vi "gentec-M-Link.Set Anticipation.vi"(0 "VISA resource In":refnum<visa-resource-name>, 2 "Enable Anticipation":bool, 5 "error in (no error)":errorcluster) -> (11 "Data Read":string, 13 "Read Timeout":bool, 14 "VISA resource Out":refnum<visa-resource-name>, 16 "Success":bool, 19 "error out":errorcluster)   [LabVIEW 2014, in "gentec-M-Link - Driver.lvlib"]
doc: "Data to write: spd0 or spd1\n\nEnables (true) or disables (false) anticipation for Thermopile Heads. Replies \"ok\"."
uses:
  gentec-M-Link - Driver.lvlib
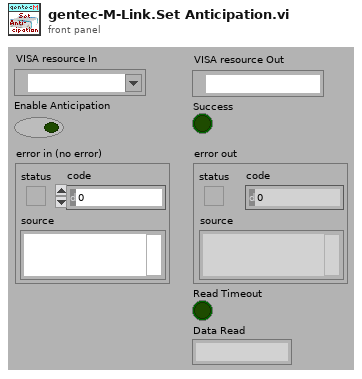
[diagram p1: front panel]
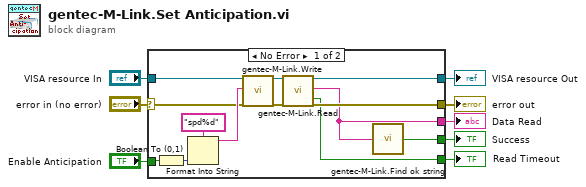
[diagram p0: block diagram]
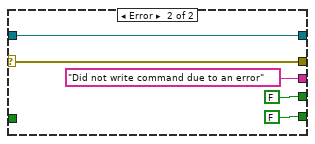
[diagram p2: hidden frame]
diagram:
  n1 = case shown="No Error" "error in (no error)" {
    selector: "error in (no error)" -> [w18 w26]
    tunnel: [w20 w26] -> w7
    tunnel: "VISA resource In" -> [w17 w25]
    tunnel: [w14 FALSE ("Found")] -> w5
    tunnel: [w13 w25] -> w4
    tunnel: "Enable Anticipation" -> [w12 _]
    tunnel: [w10 "Did not write command due to an error" ("Data Read")] -> w2
    tunnel: [w9 FALSE ("Read Timeout")] -> w1
    frame No Error {
      n2 = Boolean To (0,1)(Boolean=w12) -> (0, 1=w11:i16)
      n3 = Format Into String(format string="spd%d", w11) -> (resulting string=w19:string)  [unwired: 2 in, 1 out]
      n4 = call "gentec-M-Link.Write.vi"("VISA resource (In)"=w17, "Data To Write"=w19, "error in (no error)"=w18) -> ("VISA resource (Out)"=w16:refnum<visa-resource-name>, "error out"=w15:errorcluster)  [unwired: 14 in, 1 out]
      n5 = call "gentec-M-Link.Read.vi"("VISA resource (In)"=w16, "error in (no error)"=w15) -> ("VISA resource (Out)"=w13:refnum<visa-resource-name>, "Data Read"=w10:string, "Read Timeout"=w9:bool, "error out"=w20:errorcluster)  [unwired: 13 in, 1 out]
      n6 = call "gentec-M-Link.Find ok string.vi"("string"=w10) -> ("Found"=w14:bool)
    }
    frame Error {
    }
  }
  "error out" <- w7
  "Success" <- w5
  "VISA resource Out" <- w4
  "Data Read" <- w2
  "Read Timeout" <- w1
